vi "Server - Main.vi"() -> ()   [LabVIEW 2020]
uses:
  shared/controls/Ports to Check.ctl
  shared/controls/States.ctl
panel:
  in  "stop":bool
  in  "cRIO Client Address":string="127.0.0.1"
  out "error out":errorcluster
  out "Ports to Check":T1={"TCP Ports"=[82, 482, 5672, 6343, 8002, 49580, 3580, 80, 22, 44516, 52725, 8080], "UDP Ports"=[5353, 44515, 44525]}
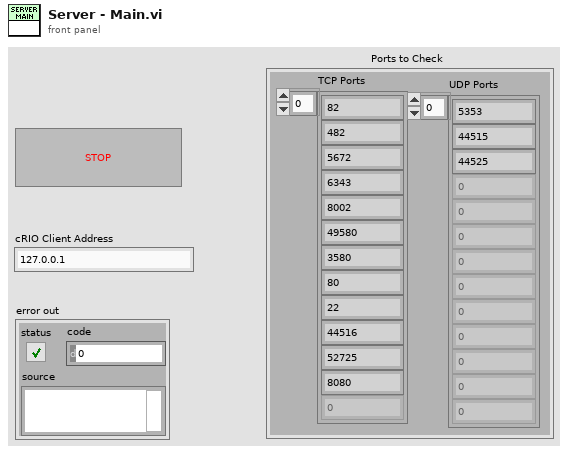
[diagram p1: front panel]
types:
  T1 = typedef "Ports to Check.ctl" = cluster{"TCP Ports":u32[], "UDP Ports":u32[]}
  T2 = typedef "States.ctl" = enum16{"Initialize", "Idle", "Establish Connection", "Start Test", "TCP Tests", "UDP Tests", "Test Complete", "View Results", "Log Results", "Edit Configuration", "Stop"}
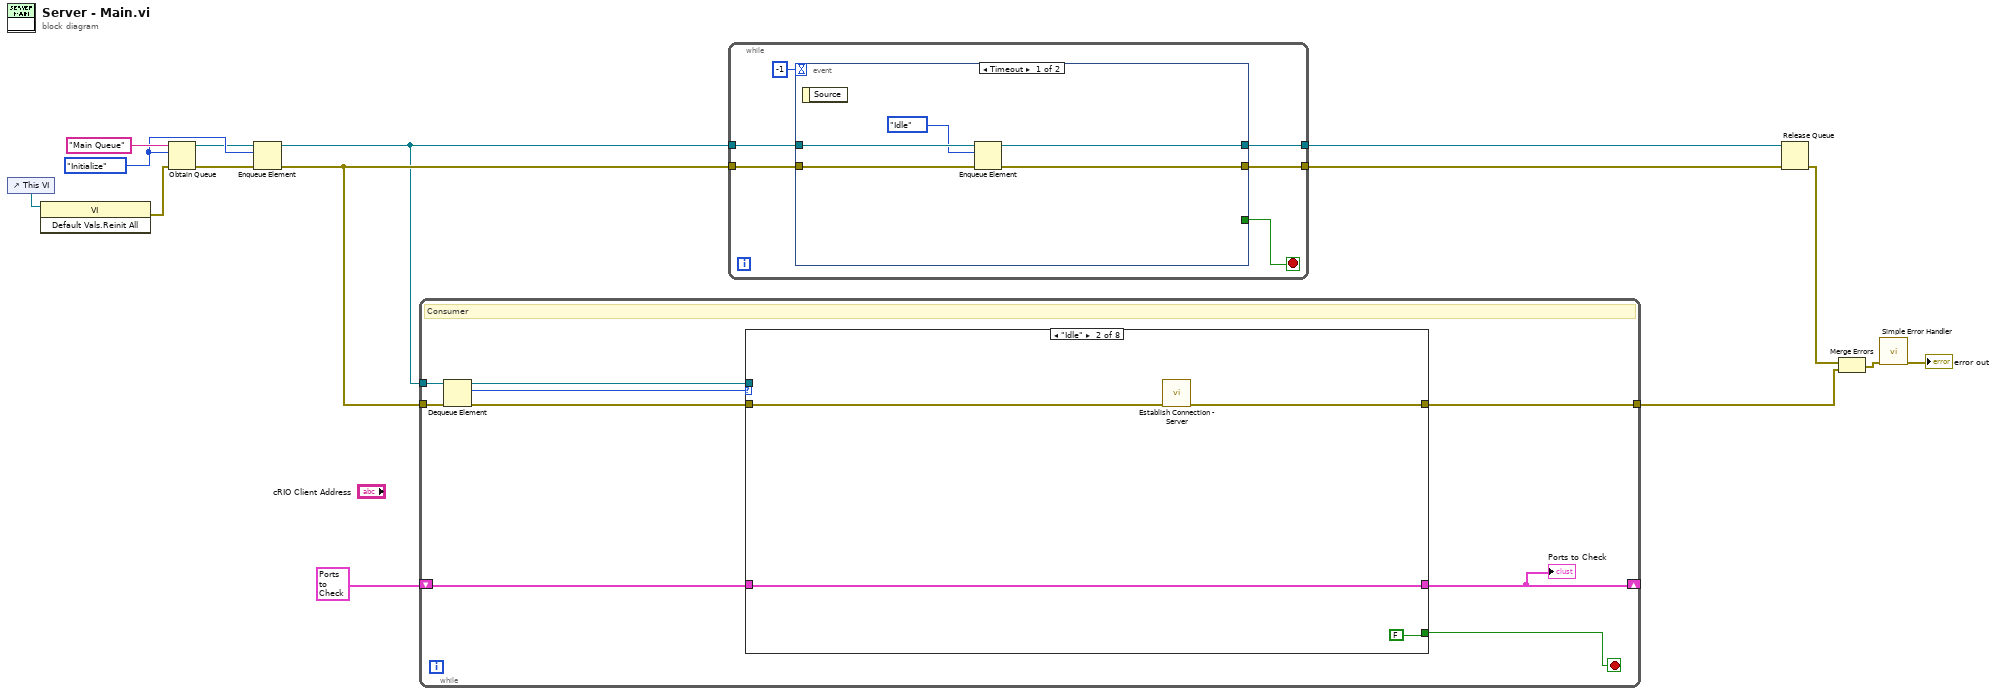
[diagram p0: block diagram]
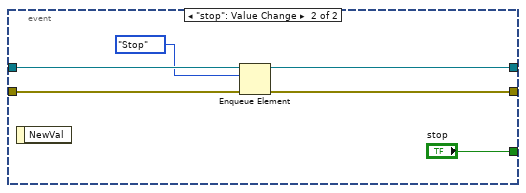
[diagram p2: hidden frame]
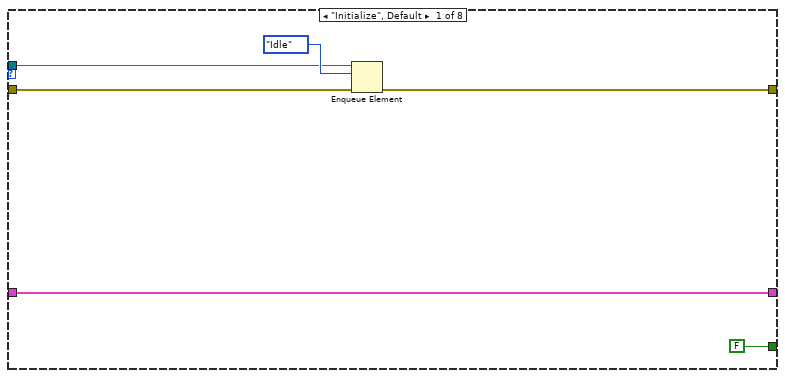
[diagram p3: hidden frame]
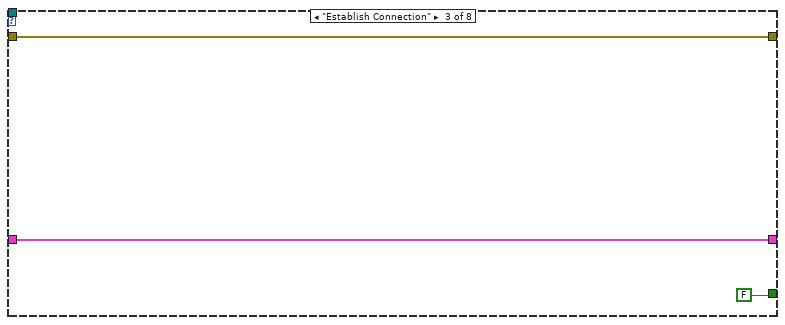
[diagram p4: hidden frame]
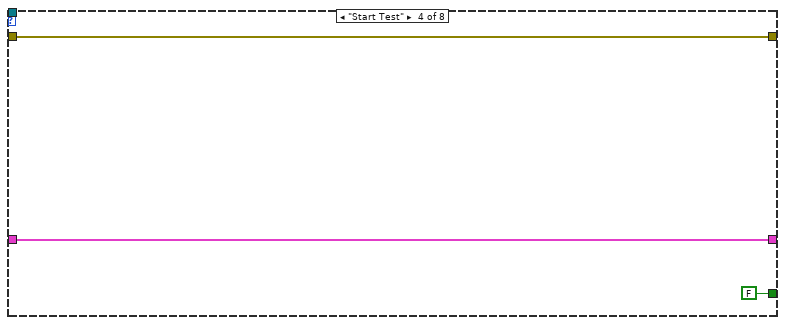
[diagram p5: hidden frame]
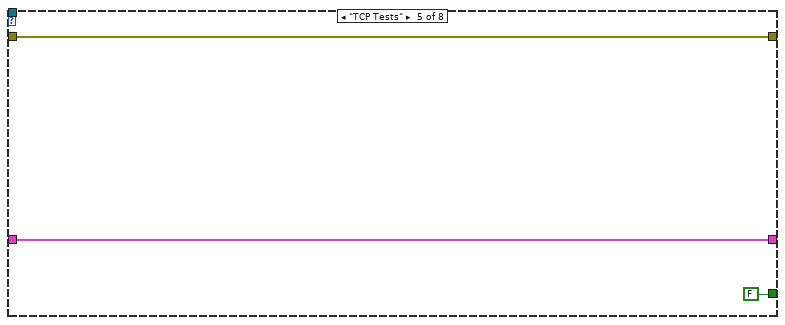
[diagram p6: hidden frame]
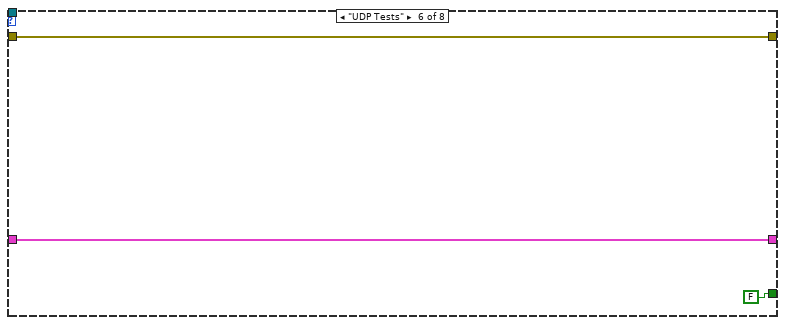
[diagram p7: hidden frame]
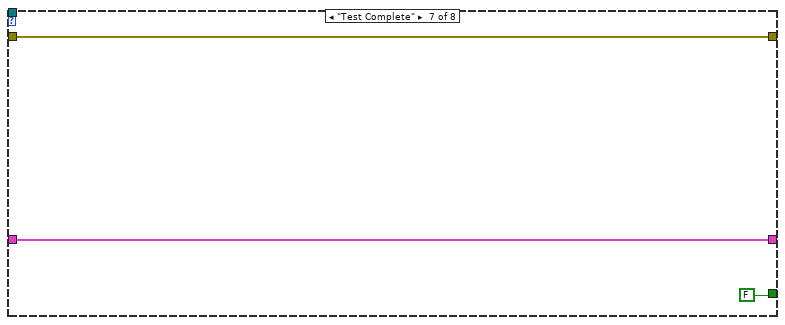
[diagram p8: hidden frame]
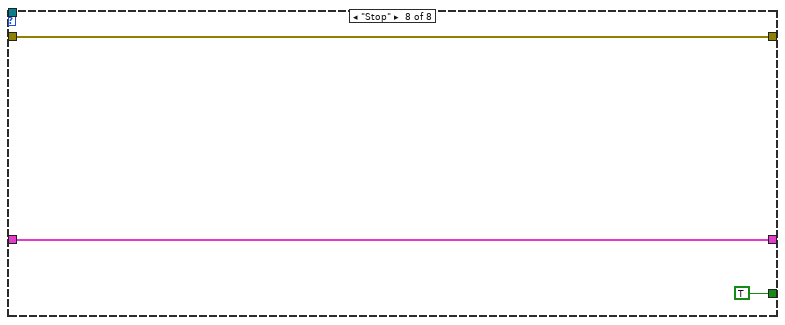
[diagram p9: hidden frame]
diagram:
  w5 = States."Initialize" ("States")
  n1 = control-ref of="This VI"() -> (w8:refnum<vi>)
  n2 = invoke class="VI" method="Default Vals.Reinit All"(reference=w8) -> (error out=w7:errorcluster)  [unwired: 2 in, 2 out]
  n3 = Obtain Queue(name (unnamed)="Main Queue", element data type=w5, error in (no error)=w7) -> (queue out=w3:refnum<queue>, error out=w9:errorcluster)  [unwired: 2 in, 1 out]
  n4 = Enqueue Element(queue=w3, element=w5, error in (no error)=w9) -> (queue out=w4:refnum<queue>, error out=w6:errorcluster)  [unwired: 1 in, 1 out]
  n5 = while {
    tunnel: w4 -> [w24]
    tunnel: w6 -> [w23]
    shift-right: [w20] -> _
    shift-left: T1 {"TCP Ports"=[82, 482, 5672, 6343, 8002, 49580, 3580, 80, 22, 44516, 52725, 8080], "UDP Ports"=[5353, 44515, 44525]} ("Ports to Check") -> [w21]
    tunnel: [w16] -> w1
    stop <- w19 stop-if-true
    # "Consumer"
    n6 = Dequeue Element(queue=w24, error in (no error)=w23) -> (queue out=w18:refnum<queue>, element=w22:T2, error out=w17:errorcluster)  [unwired: 1 in, 1 out]
    n7 = case shown="\"Idle\"" w22 {
      tunnel: w21 -> [w30 w33 w36 w39 w42 w45 w48 w51]
      tunnel: [w30 w33 w36 w39 w42 w45 w48 w51] -> w20
      tunnel: [FALSE FALSE FALSE FALSE FALSE FALSE FALSE TRUE] -> w19
      tunnel: w18 -> [w27 _ _ _ _ _ _ _]
      tunnel: w17 -> [w26 w32 w35 w38 w41 w44 w47 w50]
      tunnel: [w25 w31 w35 w38 w41 w44 w47 w50] -> w16
      frame "Initialize", Default {
        n8 = Enqueue Element(queue=w27, element=States."Idle" ("States"), error in (no error)=w26) -> (error out=w25:errorcluster)  [unwired: 1 in, 2 out]
      }
      frame "Idle" {
        n9 = call "Establish Connection - Server.vi"("error in (no error)"=w32) -> ("error out"=w31:errorcluster)  [unwired: 9 in]
      }
      frame "Establish Connection" {
      }
      frame "Start Test" {
      }
      frame "TCP Tests" {
      }
      frame "UDP Tests" {
      }
      frame "Test Complete" {
      }
      frame "Stop" {
      }
    }
    "Ports to Check" <- w20
  }
  n10 = while {
    tunnel: w4 -> [w58]
    tunnel: [w57] -> w14
    tunnel: w6 -> [w55]
    tunnel: [w54] -> w11
    stop <- w56 stop-if-true
    n11 = event shown="[0] Timeout" {
      selector: _ -> [_ _]
      dyn-events: _ -> [_ _]
      timeout: -1 -> [_ _]
      tunnel: w58 -> [w63 w69]
      tunnel: [w62 w68] -> w57
      tunnel: [_ "stop"] -> w56
      tunnel: w55 -> [w61 w66]
      tunnel: [w60 w65] -> w54
      event Timeout {
        n12 = event-data() -> ()  [unwired: 1 in, 1 out]
        n13 = Enqueue Element(queue=w63, element=States."Idle" ("States"), error in (no error)=w61) -> (queue out=w62:refnum<queue>, error out=w60:errorcluster)  [unwired: 1 in, 1 out]
      }
      event "stop": Value Change {
        n14 = event-data() -> ()  [unwired: 1 in, 1 out]
        n15 = Enqueue Element(queue=w69, element=States."Stop" ("States"), error in (no error)=w66) -> (queue out=w68:refnum<queue>, error out=w65:errorcluster)  [unwired: 1 in, 1 out]
      }
    }
  }
  n16 = Release Queue(queue=w14, error in (no error)=w11) -> (error out=w10:errorcluster)  [unwired: 1 in, 2 out]
  n17 = Merge Errors(w10, w1) -> (w12:errorcluster)
  n18 = call <vilib>:"Simple Error Handler.vi"("error in (no error)"=w12) -> ("error out"=→"error out":errorcluster)  [unwired: 4 in, 4 out]
